vi "host_abort.vi"(8 "error in":errorcluster) -> (0 "error out":errorcluster)   [LabVIEW 2021]
uses:
  host_global_vars.vi
  <vilib>/Utility/error.llb/Error Cluster From Error Code.vi
  <vilib>/rvi/errors/niLvFpgaAdjustHostInterfaceError.vi
  <vilib>/rvi/interface/nirviReadWriteControl/nirviReadWriteControl.xnode
  FPGA Bitfiles/openlabspm_FPGATarget_fpgamain_eo-gUZR5D1g.lvbitx
  fpga/fpga_main.vi
  NiFpgaLv.dll
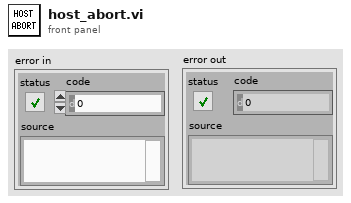
[diagram p1: front panel]
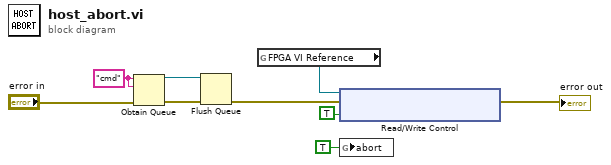
[diagram p0: block diagram]
diagram:
  w1 = "cmd" ("name (unnamed)")
  n1 = Obtain Queue(name (unnamed)=w1, element data type=w1, error in (no error)="error in") -> (queue out=w6:refnum<queue>, error out=w7:errorcluster)  [unwired: 2 in, 1 out]
  n2 = Flush Queue(queue=w6, error in (no error)=w7) -> (error out=w5:errorcluster)  [unwired: 2 out]
  n3 = global read "host_global_vars.vi" "FPGA VI Reference"() -> (w9:refnum<k20>)
  n4 = xnode "Read/Write Control"("FPGA VI Reference In"=w9, "error in"=w5, "Abort"=TRUE ("scan?")) -> ("error out"=→"error out":errorcluster)  [unwired: 1 out]
  n5 = global write "host_global_vars.vi" "abort"(TRUE ("abort")) -> ()
